vi "Get Base.vi"(8 "error in":errorcluster, 11 "Default Value":string) -> (0 "error out":errorcluster, 2 "Number Base":u8, 3 "Default Value (dup)":string)   [LabVIEW 2020, in "CANopen.lvlib"]
doc: "Return number base of a string (10 for desimal, 16 for hex and 8 for octal)"
uses:
  CANopen.lvlib
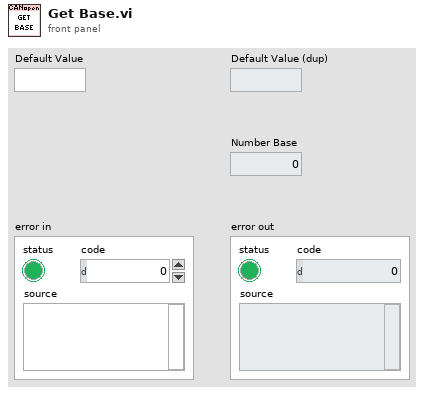
[diagram p1: front panel]
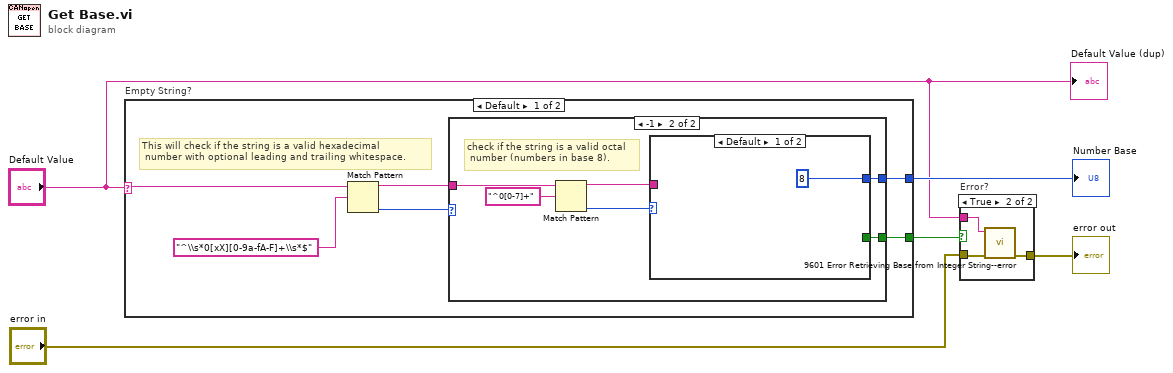
[diagram p0: block diagram]
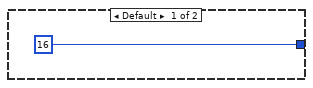
[diagram p3: hidden frame]
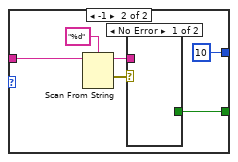
[diagram p4: hidden frame]
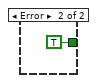
[diagram p5: hidden frame]
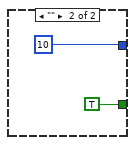
[diagram p6: hidden frame]
diagram:
  n1 = case "Empty String?" shown="Default" "Default Value" {
    selector: "Default Value" -> [w11 _]
    tunnel: [w8 u8 10] -> w5
    tunnel: [w6 TRUE] -> w3
    frame Default {
      # "This will check if the string is a valid hexadecimal\n number with optional leading and trailing whitespace."
      n2 = Match Pattern(string=w11, regular expression="^\\s*0[xX][0-9a-fA-F]+\\s*$") -> (before substring=w7:string, offset past match=w9:i32)  [unwired: 1 in, 2 out]
      n3 = case shown="-1" w9 {
        tunnel: [u8 16 w16] -> w8
        tunnel: w7 -> [_ w18]
        tunnel: [_ w13] -> w6
        frame Default {
        }
        frame -1 {
          # "check if the string is a valid octal\n number (numbers in base 8)."
          n4 = Match Pattern(string=w18, regular expression="^0[0-7]+") -> (before substring=w14:string, offset past match=w15:i32)  [unwired: 1 in, 2 out]
          n5 = case shown="Default" w15 {
            tunnel: [u8 8 u8 10] -> w16
            tunnel: w14 -> [_ w25]
            tunnel: [_ w21] -> w13
            frame Default {
            }
            frame -1 {
              n6 = Scan From String(format string="%d", input string=w25) -> (remaining string=w22:string, error out=w23:errorcluster)  [unwired: 4 in, 1 out]
              n7 = case shown="No Error" w23 {
                tunnel: w22 -> [_ _]
                tunnel: [_ TRUE] -> w21
                frame No Error {
                }
                frame Error {
                }
              }
            }
          }
        }
      }
    }
    frame "" {
    }
  }
  "Number Base" <- w5
  n8 = case "Error?" shown="True" w3 {
    tunnel: [w29 w32] -> w4
    tunnel: "error in" -> [w29 w31]
    tunnel: "Default Value" -> [_ w30]
    frame False {
    }
    frame True {
      n9 = call "9601 Error Retrieving Base from Integer String--error.vi"("error in"=w31, "Integer String"=w30) -> ("error out"=w32:errorcluster)  [unwired: 9 in]
    }
  }
  "error out" <- w4
  "Default Value (dup)" <- "Default Value"
